vi "Wire Event Data Out.vi"(8 "error in (no error)":errorcluster, 9 "Event Data Names":string[](array[string]), 10 "Event Data":refnum<vi>[](array[refnum]), 11 "Diagram in":refnum<vi>) -> (0 "error out":errorcluster, 3 "Diagram out":refnum<vi>)   [LabVIEW 2015, in "Scripting.lvlib"]
uses:
  Scripting.lvlib
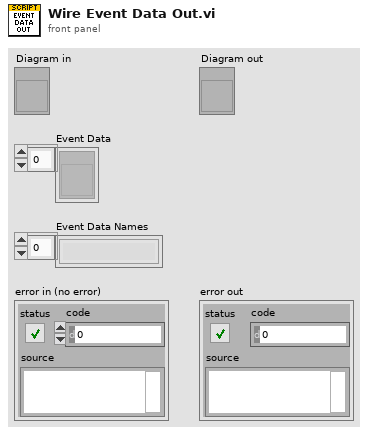
[diagram p1: front panel]
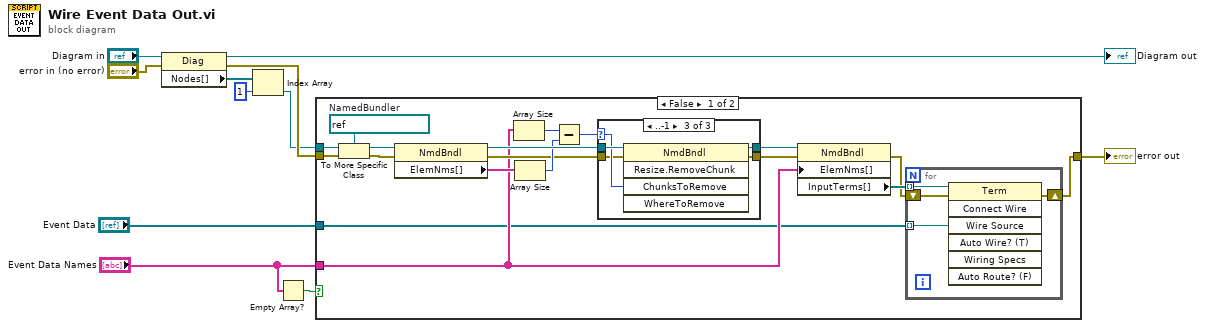
[diagram p0: block diagram]
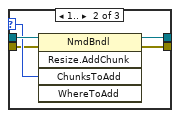
[diagram p3: hidden frame]
diagram:
  n1 = property class="Diag"(reference="Diagram in", error in="error in (no error)") -> (reference out=→"Diagram out":refnum<vi>, error out=w10:errorcluster, "Nodes[]"=w4:refnum<vi>[])
  n2 = Index Array(array=w4, index=1) -> (element=w6:refnum<vi>)
  n3 = Empty Array?(array="Event Data Names") -> (empty?=w8:bool)
  n4 = case shown="False" w8 {
    tunnel: w6 -> [w29 _]
    tunnel: w10 -> [w28 w46]
    tunnel: "Event Data Names" -> [w16 _]
    tunnel: [w12 w46] -> w11
    tunnel: "Event Data" -> [w14 _]
    frame False {
      w27 = refnum<vi> refnum  # NamedBundler
      n5 = To More Specific Class(target class=w27, reference=w29, error in=w28) -> (specific class reference=w21:refnum<vi>, error out=w18:errorcluster)
      n6 = property class="NmdBndl"(reference=w21, error in=w18) -> (reference out=w26:refnum<vi>, error out=w17:errorcluster, "ElemNms[]"=w25:string[])
      n7 = Array Size(array=w16) -> (size(s)=w23:i32)
      n8 = Array Size(array=w25) -> (size(s)=w24:i32)
      n9 = Subtract(x=w23, y=w24) -> (x-y=w22:i32)
      n10 = case shown="..-1" w22 {
        selector: w22 -> [_ w39 w44]
        tunnel: w26 -> [w35 w40 w45]
        tunnel: [w35 w38 w43] -> w20
        tunnel: w17 -> [w34 w37 w41]
        tunnel: [w34 w36 w42] -> w19
        frame 0 {
        }
        frame 1.. {
          n11 = invoke class="NmdBndl" method="Resize.AddChunk"(reference=w40, error in=w37, "ChunksToAdd"=w39) -> (reference out=w38:refnum<vi>, error out=w36:errorcluster)  [unwired: 2 in, 3 out]
        }
        frame ..-1 {
          n12 = invoke class="NmdBndl" method="Resize.RemoveChunk"(reference=w45, error in=w41, "ChunksToRemove"=w44) -> (reference out=w43:refnum<vi>, error out=w42:errorcluster)  [unwired: 2 in, 3 out]
        }
      }
      n13 = property class="NmdBndl"(reference=w20, error in=w19, "ElemNms[]"=w16) -> (error out=w13:errorcluster, "InputTerms[]"=w15:refnum<vi>[])  [unwired: 1 out]
      n14 = for {
        tunnel: w15 -> [w33] mode=indexing
        tunnel: w14 -> [w32] mode=indexing
        shift-right: [w30] -> w12
        shift-left: w13 -> [w31]
        n15 = invoke class="Term" method="Connect Wire"(reference=w33, error in=w31, "Wire Source"=w32) -> (error out=w30:errorcluster)  [unwired: 4 in, 6 out]
      }
    }
    frame True {
    }
  }
  "error out" <- w11
